vi "EJ 4.2.4.vi"() -> ()   [LabVIEW 2013]
uses:
  <vilib>/sound2/lvsound2.llb/Sound Input Read (DBL).vi
panel:
  out "Boolean":bool
  out "Numeric":dbl
  in  "Frecuencia":dbl
  in  "stop":bool
  in  "Cluster":T1
  out "Waveform Graph":dbl[](graph)
  in  "Buffer de lectura":dbl=11025.0
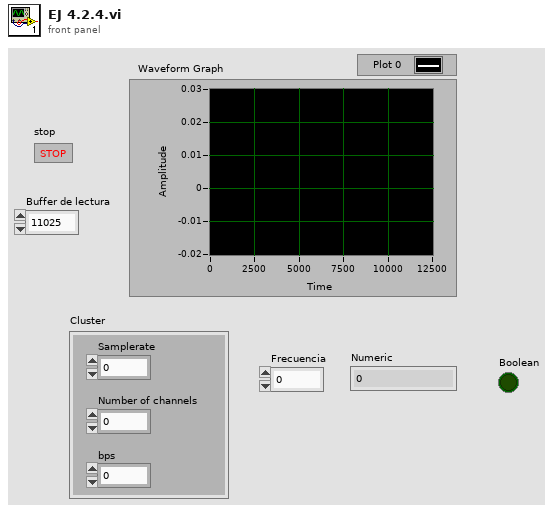
[diagram p1: front panel]
types:
  T1 = cluster{"Samplerate":dbl, "Number of channels":dbl, "bps":dbl}
  T2 = typedef "Sound Input Task ID.ctl" = u32
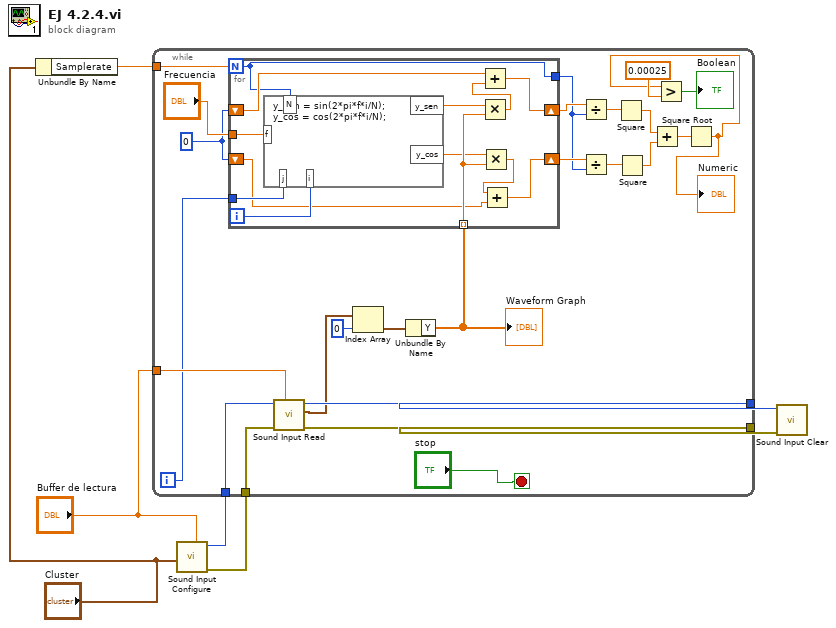
[diagram p0: block diagram]
diagram:
  n1 = Unbundle By Name("Cluster") -> ("Samplerate"=w1:dbl)
  n2 = call <vilib>:"Sound Input Configure.vi"("number of samples/ch"="Buffer de lectura", "sound format"="Cluster") -> ("error out"=w7:errorcluster, "task ID"=w5:T2)  [unwired: 8 in]
  n3 = while {
    tunnel: w7 -> [w30]
    tunnel: [w29] -> w6
    tunnel: w5 -> [w31]
    tunnel: [w32] -> w4
    tunnel: "Buffer de lectura" -> [w28]
    tunnel: w1 -> [w8]
    i -> [w20]
    stop <- "stop" stop-if-true
    w21 = 0
    n4 = call-poly <vilib>:"Sound Input Read.vi"("number of samples/ch"=w28, "error in (no error)"=w30, "task ID"=w31) -> ("error out"=w29:errorcluster, "data"=w27:waveform(dbl)[], "task ID out"=w32:T2)  [unwired: 6 in]
    n5 = Index Array(array=w27, index=0) -> (element=w25:waveform(dbl))
    n6 = Unbundle By Name(w25) -> ("Y"=w22:dbl[])
    "Waveform Graph" <- w22
    n7 = for {
      N: w8 -> [w33]
      tunnel: "Frecuencia" -> [w45]
      tunnel: w22 -> [w43] mode=indexing
      shift-right: [w38] -> w13
      shift-left: w21 -> [w37]
      shift-right: [w34] -> w14
      shift-left: w21 -> [w35]
      tunnel: w20 -> [w40]
      tunnel: [w33] -> w12
      i -> [w44]
      n8 = formula code="y_sen = sin(2*pi*f*i/N);\ny_cos = cos(2*pi*f*i/N);"("i"=w44, "j"=w40, "f"=w45, "N"=w33) -> ("y_sen"=w41:dbl, "y_cos"=w42:dbl)
      n9 = Multiply(x=w41, y=w43) -> (x*y=w39:dbl)
      n10 = Add(x=w37, y=w39) -> (x+y=w38:dbl)
      n11 = Multiply(x=w42, y=w43) -> (x*y=w36:dbl)
      n12 = Add(x=w36, y=w35) -> (x+y=w34:dbl)
    }
    n13 = Divide(x=w13, y=w12) -> (x/y=w19:dbl)
    n14 = Divide(x=w14, y=w12) -> (x/y=w18:dbl)
    n15 = Square(x=w19) -> (x^2=w17:dbl)
    n16 = Square(x=w18) -> (x^2=w16:dbl)
    n17 = Add(x=w17, y=w16) -> (x+y=w15:dbl)
    n18 = Square Root(x=w15) -> (sqrt(x)=w10:dbl)
    "Numeric" <- w10
    n19 = Greater?(x=w10, y=0.00025) -> (0:→"Boolean":bool)
  }
  n20 = call <vilib>:"Sound Input Clear.vi"("error in (no error)"=w6, "task ID"=w4) -> ()  [unwired: 9 in, 1 out]
